vi "Initialize.vi"(8 "error in":errorcluster, 11 "Plugin in":refnum<class "Waterfall.lvclass">) -> (0 "error out":errorcluster, 3 "Plugin out":refnum<class "Waterfall.lvclass">)   [LabVIEW 2024, in "Waterfall.lvlib" / "Waterfall.lvclass"]
uses:
  Waterfall.lvclass
  C:/Program Files/National Instruments/LabVIEW 2024/vi.lib/FlexLogger/SDK/PluginSDK.lvlibp/PEFClasses/SDK/Plugin/Plugin.lvclass
  <vilib>/FlexLogger/SDK/PluginSDK.lvlibp/PEFClasses/SDK/Processing Element/Timing Parameters.ctl
  <vilib>/FlexLogger/SDK/PluginSDK.lvlibp/PEFClasses/SDK/Processing Element/Timing Method.ctl
  <vilib>/FlexLogger/SDK/PluginSDK.lvlibp/PEFClasses/SDK/System Interface/Resampling Mode.ctl
  Waterfall Global.vi
  <vilib>/FlexLogger/SDK/PluginSDK.lvlibp/PEFClasses/SDK/Plugin/ParameterAccess/Write Single Channel.vi
  <vilib>/FlexLogger/SDK/PluginSDK.lvlibp/PEFClasses/SDK/Plugin/ParameterAccess/Write DBL.vi
  <vilib>/FlexLogger/SDK/PluginSDK.lvlibp/PEFClasses/SDK/Plugin/ParameterAccess/Write Enum.vi
  <vilib>/FlexLogger/SDK/PluginSDK.lvlibp/PEFClasses/SDK/Plugin/ParameterAccess/Write I32.vi
  <vilib>/FlexLogger/SDK/PluginSDK.lvlibp/PEFClasses/SDK/Plugin/ParameterAccess/Write Command.vi
  <vilib>/FlexLogger/SDK/PluginSDK.lvlibp/PEFClasses/SDK/Plugin/Plugin.lvclass
  C:/Program Files/National Instruments/LabVIEW 2024/vi.lib/FlexLogger/SDK/PluginSDK.lvlibp/PEFClasses/SDK/Processing Element/Processing Element.lvclass
  C:/Users/Administrator/Documents/LabVIEW Projects/FlexLogger IO Plug-ins/Waterfall/Waterfall.lvclass
  <vilib>/FlexLogger/SDK/PluginSDK.lvlibp/PEFClasses/SDK/Processing Element/Processing Element.lvclass
  <vilib>/FlexLogger/SDK/PluginSDK.lvlibp/PEFClasses/SDK/System Interface/System Interface.lvclass
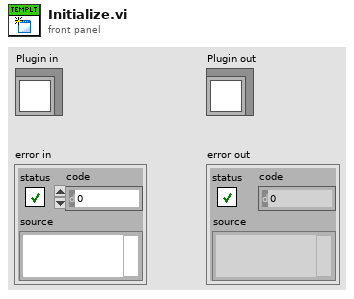
[diagram p1: front panel]
types:
  T1 = typedef "PluginSDK.lvlibp/System Interface.lvclass/Resampling Mode.ctl" = enum16{"No Resampling", "Custom Rate", "Maximum Rate", "Minimum Rate"}
  T2 = typedef "PluginSDK.lvlibp/Processing Element.lvclass/Timing Parameters.ctl" = cluster{"Timing Method":T3, "Timing Period (ms)":i32}
  T3 = typedef "PluginSDK.lvlibp/Processing Element.lvclass/Timing Method.ctl" = enum16{"Periodic", "Immediate", "On Data Ready", "Triggered"}
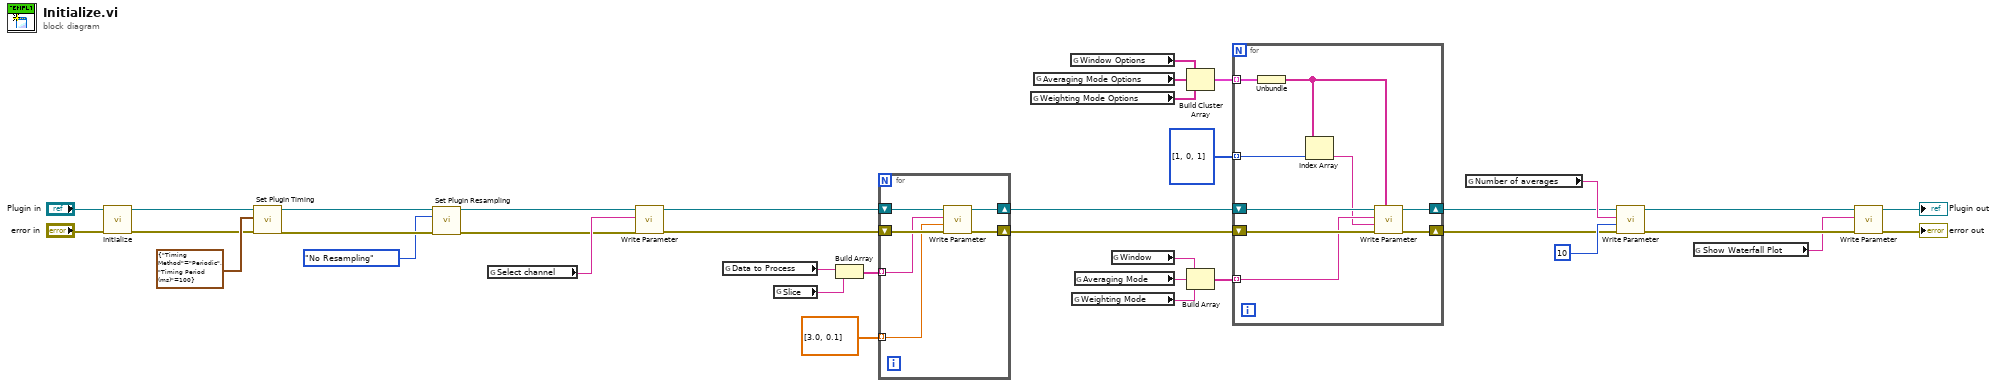
[diagram p0: block diagram]
diagram:
  n1 = call-parent "Initialize.vi"("error in (no error)"="error in", "Plugin in"="Plugin in") -> ("error out"=w14:errorcluster, "Plugin out"=w15:refnum<class "Waterfall.lvclass">)  [unwired: 8 in]
  n2 = call <vilib>:"Set Plugin Timing.vi"("error in (no error)"=w14, "Timing Parameters"=T2 {"Timing Method"=enum."Periodic", "Timing Period (ms)"=100}, "Plugin in"=w15) -> ("error out"=w11:errorcluster, "Plugin out"=w13:refnum<class "Waterfall.lvclass">)  [unwired: 7 in]
  n3 = call <vilib>:"Set Plugin Resampling.vi"("Plugin in"=w13, "Resampling Mode"=Resampling_Mode."No Resampling", "error in (no error)"=w11) -> ("Plugin out"=w12:refnum<class "Waterfall.lvclass">, "error out"=w10:errorcluster)  [unwired: 11 in]
  n4 = global read "Waterfall Global.vi" "Select channel"() -> (w35:string)
  n5 = call-poly <vilib>:"Write Parameter.vi"("error in (no error)"=w10, "Name (Unique Channel Identifier)"=w35, "Plugin in"=w12) -> ("error out"=w5:errorcluster, "Plugin out"=w6:refnum<class "Waterfall.lvclass">)  [unwired: 7 in]
  n6 = global read "Waterfall Global.vi" "Data to Process"() -> (w4:string)
  n7 = global read "Waterfall Global.vi" "Slice"() -> (w3:string)
  n8 = Build Array(w4, w3) -> (w7:string[])
  n9 = for {
    shift-right: [w42] -> w2
    shift-left: w6 -> [w43]
    shift-right: [w40] -> w1
    shift-left: w5 -> [w41]
    tunnel: dbl[] [3.0, 0.1] -> [w38] mode=indexing
    tunnel: w7 -> [w39] mode=indexing
    n10 = call-poly <vilib>:"Write Parameter.vi"("error in (no error)"=w41, "Value"=w38, "Name"=w39, "Plugin in"=w43) -> ("error out"=w40:errorcluster, "Plugin out"=w42:refnum<class "Waterfall.lvclass">)  [unwired: 6 in]
  }
  n11 = global read "Waterfall Global.vi" "Weighting Mode Options"() -> (w21:string[])
  n12 = global read "Waterfall Global.vi" "Averaging Mode Options"() -> (w26:string[])
  n13 = global read "Waterfall Global.vi" "Window Options"() -> (w27:string[])
  n14 = global read "Waterfall Global.vi" "Weighting Mode"() -> (w20:string)
  n15 = global read "Waterfall Global.vi" "Averaging Mode"() -> (w22:string)
  n16 = global read "Waterfall Global.vi" "Window"() -> (w23:string)
  n17 = Build Cluster Array(w27, w26, w21) -> (w25:cluster{"Weighting Mode Options":string[]}[])
  n18 = Build Array(w23, w22, w20) -> (w19:string[])
  n19 = for {
    tunnel: w25 -> [w48] mode=indexing
    shift-right: [w51] -> w18
    shift-left: w2 -> [w52]
    shift-right: [w49] -> w17
    shift-left: w1 -> [w50]
    tunnel: i32[] [1, 0, 1] -> [w46] mode=indexing
    tunnel: w19 -> [w45] mode=indexing
    n20 = Unbundle(w48) -> ("Weighting Mode Options"=w47:string[])
    n21 = Index Array(array=w47, index=w46) -> (element=w44:string)
    n22 = call-poly <vilib>:"Write Parameter.vi"("Possible Values"=w47, "error in (no error)"=w50, "Current Value"=w44, "Name"=w45, "Plugin in"=w52) -> ("error out"=w49:errorcluster, "Plugin out"=w51:refnum<class "Waterfall.lvclass">)  [unwired: 5 in]
  }
  n23 = global read "Waterfall Global.vi" "Number of averages"() -> (w33:string)
  n24 = call-poly <vilib>:"Write Parameter.vi"("error in (no error)"=w17, "Value"=10, "Name"=w33, "Plugin in"=w18) -> ("error out"=w30:errorcluster, "Plugin out"=w32:refnum<class "Waterfall.lvclass">)  [unwired: 6 in]
  n25 = global read "Waterfall Global.vi" "Show Waterfall Plot"() -> (w28:string)
  n26 = call-poly <vilib>:"Write Parameter.vi"("error in (no error)"=w30, "Name"=w28, "Plugin in"=w32) -> ("error out"=→"error out":errorcluster, "Plugin out"=→"Plugin out":refnum<class "Waterfall.lvclass">)  [unwired: 7 in]
